vi "Read APU 1.3 Position.vi"(8 "error in (no error)":errorcluster, 11 "APU in":refnum<class "APU.lvclass">) -> (0 "error out":errorcluster, 1 "cycle angle":dbl, 2 "crank angle":dbl, 3 "APU out":refnum<class "APU.lvclass">)   [LabVIEW 2013, in "APU.lvclass"]
uses:
  APU.lvclass
  Engine Simulation IP.lvclass/Engine Simulation IP.ctl
  APU.lvclass/APU.ctl
  <vilib>/rvi/interface/common/niFpgaWaitOnOcc.vi
  <vilib>/Utility/error.llb/Error Cluster From Error Code.vi
  <vilib>/rvi/errors/niLvFpgaAdjustHostInterfaceError.vi
  <vilib>/rvi/interface/nirviReadWriteControl/nirviReadWriteControl.xnode
  Engine Simulation IP.lvclass
  NiFpgaLv.dll
  <vilib>/rvi/interface/Simulation/niFpgaSimulationCallBeginRW.vi
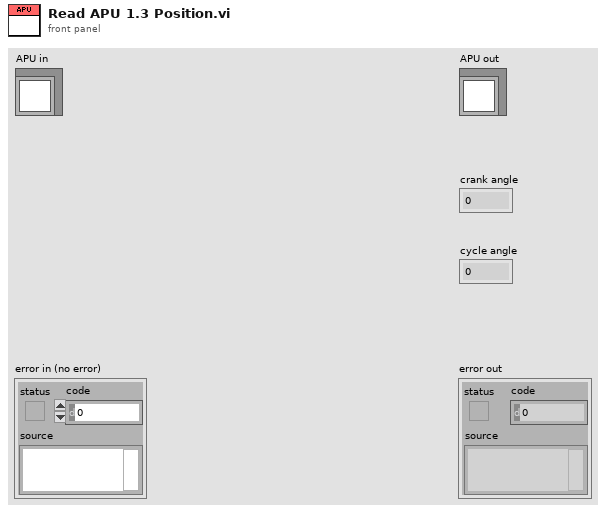
[diagram p1: front panel]
types:
  T1 = typedef "Engine Simulation Session.lvclass/Bitfile Major Version.ctl" = enum16{"1.0", "1.1", "1.2", "1.3"}
  T2 = cluster{"crank":u16, "cycle":u16, "actual speed":fxp<+/-,23,2>}
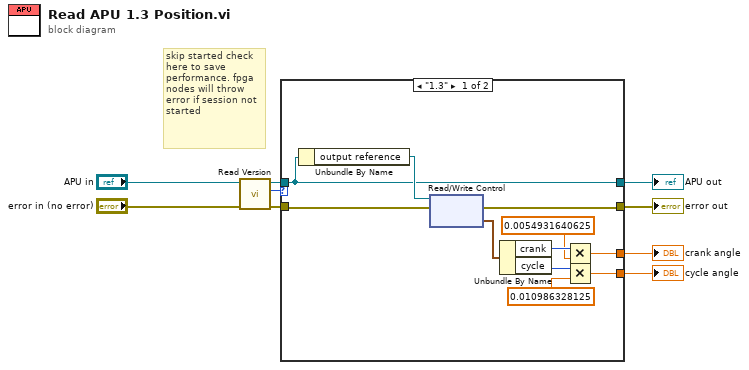
[diagram p0: block diagram]
diagram:
  # "skip started check here to save performance. fpga nodes will throw error if session not started"
  n1 = call "Read Version.vi"("error in (no error)"="error in (no error)", "Engine Simulation IP in"="APU in") -> ("error out"=w3:errorcluster, "version"=w2:T1, "Engine Simulation IP out"=w1:refnum<class "APU.lvclass">)  [unwired: 7 in]
  n2 = case shown="\"1.3\"" w2 {
    tunnel: [w20 w22] -> w8
    tunnel: w3 -> [w19 w22]
    tunnel: w1 -> [w17 w21]
    tunnel: [w17 w21] -> w6
    tunnel: [w12 _] -> w5
    tunnel: [w10 _] -> w4
    frame "1.3" {
      n3 = Unbundle By Name(w17) -> ("output reference"=w18:refnum<k20>)
      n4 = xnode "Read/Write Control"("FPGA VI Reference In"=w18, "error in"=w19) -> ("error out"=w20:errorcluster, "Value"=w16:T2)  [unwired: 1 out]
      n5 = Unbundle By Name(w16) -> ("crank"=w14:u16, "cycle"=w15:u16)
      n6 = Multiply(x=w14, y=0.0054931640625) -> (x*y=w12:dbl)
      n7 = Multiply(x=w15, y=0.010986328125) -> (x*y=w10:dbl)
    }
    frame Default {
      # "#todo throw wrong version error"
    }
  }
  "error out" <- w8
  "APU out" <- w6
  "crank angle" <- w5
  "cycle angle" <- w4
